vi "niRFUtil WFM Parse Waveform - Duration (complex wfm).vi"(3 "Duration (Inf)":dbl=inf format="%^.6e", 4 "Start (-Inf)":dbl=-inf format="%^.6e", 5 "Waveform In":T1 {"y" format="%.2f"; "dx" format="%^.2e"; "x0" format="%^.2e"}) -> (2 "Waveform Out":T1 {"y" format="%.2f"; "dx" format="%^.2e"; "x0" format="%^.2e"})   [LabVIEW 2016, in "niRFUtil.lvlib"]
doc: "(c) Copyright 2006, National Instruments, Inc. This VI may not be duplicated, sold, or distributed without written consent from National Instruments."
uses:
  niRFUtil.lvlib
  Includes/niRFUtil INC Complex Waveform.ctl
  Includes/niRFUtil INC Complex Array.ctl
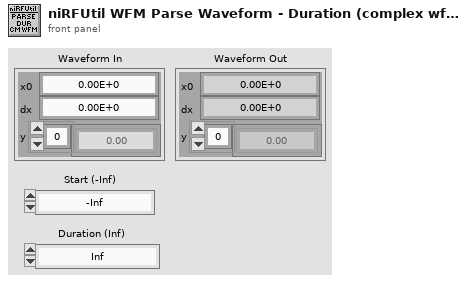
[diagram p1: front panel]
types:
  T1 = typedef "niRFUtil.lvlib/niRFUtil INC Complex Waveform.ctl" = cluster{"x0":dbl, "dx":dbl, "y":T2}
  T2 = typedef "niRFUtil.lvlib/niRFUtil INC Complex Array.ctl" = csg[]
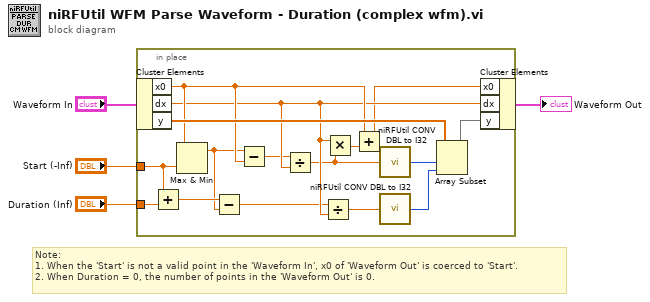
[diagram p0: block diagram]
diagram:
  # "Note:\n1. When the 'Start' is not a valid point in the 'Waveform In', x0 of 'Waveform Out' is coerced to 'Start'.\n2. When Duration = 0, the number of points in the 'Waveform Out' is 0."
  n1 = in-place {
    in-place-border: "Start (-Inf)" -> [w12]
    in-place-border: "Duration (Inf)" -> [w13]
    n2 = in-place-cluster #1("Waveform In") -> ("x0"=w18:dbl, "dx"=w16:dbl, "y"=w19:T2)
    n3 = Add(x=w12, y=w13) -> (x+y=w11:dbl)
    n4 = Max & Min(x=w18, y=w12) -> (max(x,y)=w10:dbl)  [unwired: 1 out]
    n5 = Subtract(x=w11, y=w10) -> (x-y=w9:dbl)
    n6 = Subtract(x=w10, y=w18) -> (x-y=w14:dbl)
    n7 = Divide(x=w14, y=w16) -> (x/y=w8:dbl)
    n8 = Divide(x=w9, y=w16) -> (x/y=w6:dbl)
    n9 = Multiply(x=w16, y=w8) -> (x*y=w20:dbl)
    n10 = Add(x=w18, y=w20) -> (x+y=w15:dbl)
    n11 = call "niRFUtil CONV DBL to I32.vi"("Numeric (DBL)"=w8) -> ("Numeric (I32)"=w7:i32)  [unwired: 14 in]
    n12 = call "niRFUtil CONV DBL to I32.vi"("Numeric (DBL)"=w6) -> ("Numeric (I32)"=w5:i32)  [unwired: 14 in]
    n13 = Array Subset(array=w19, index=w7, length=w5) -> (w17:T2)
    n14 = in-place-cluster #1("x0"=w15, "dx"=w16, "y"=w17) -> (→"Waveform Out":T1)
  }
